vi "OP30A_Data.vi"() -> (0 "OP20_HOSE_TEST":T1)   [LabVIEW 2020]
panel:
  in  "[Constriction_Pr_Diff]":dbl
  in  "[Constriction_Act_Pr]":dbl
  in  "[Constriction_Diff_LL]":dbl
  in  "[Constriction_Diff_HL]":dbl
  in  "[Constriction_Result]":dbl
  in  "[Constriction_Test_Time]":dbl
  in  "[HP_STS]":dbl
  in  "[PRESSURE_FILL_ACT":dbl
  in  "[PRESSURE_DROP]":dbl
  in  "[PRESSURE_DROP_MAX]":dbl
  in  "[PRESSURE_FILL_LL]":dbl
  in  "[PRESSURE_FILL_HL]":dbl
  in  "[FILL_TIME]":dbl
  in  "[STAB_TIME]":dbl
  in  "[TEST_TIME]":dbl
  in  "[CT]":dbl
  out "error out":errorcluster
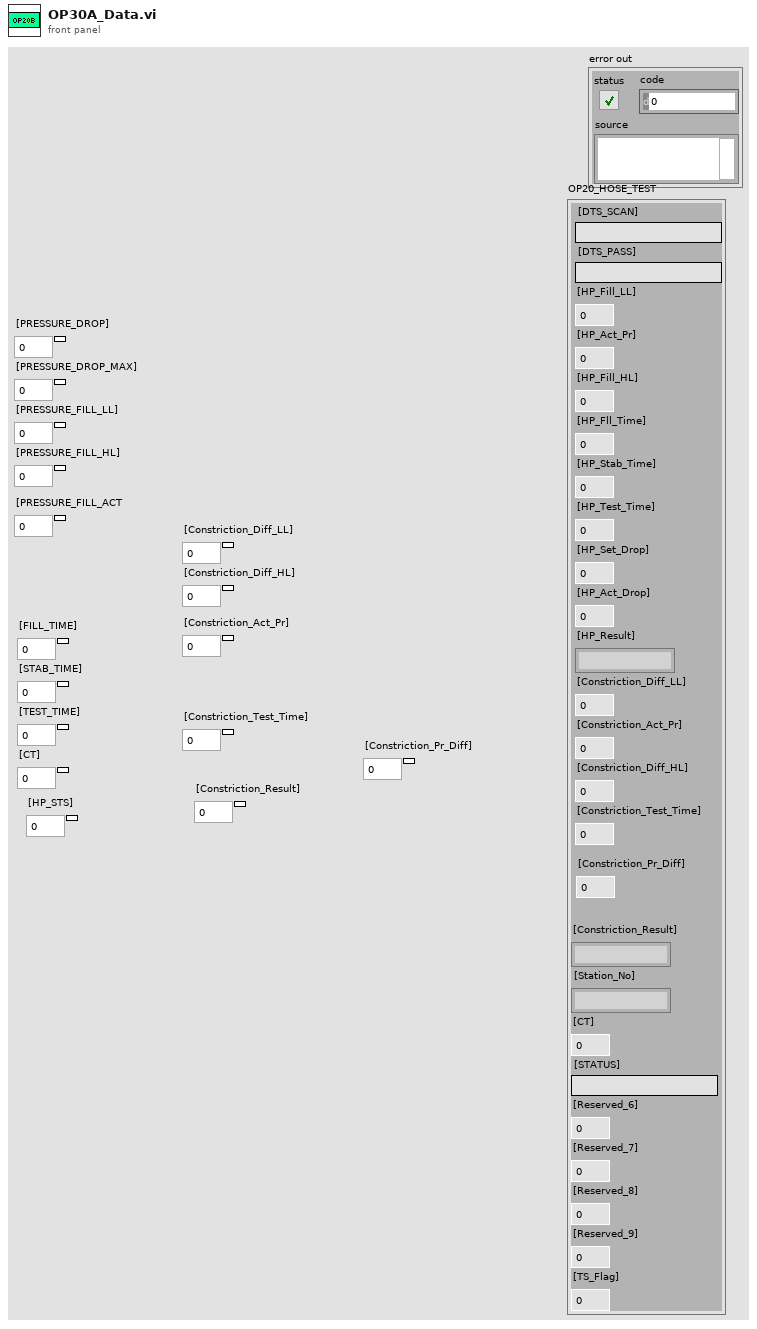
[diagram p1: front panel]
types:
  T1 = cluster{"[DTS_SCAN]":string, "[DTS_PASS]":string, "[HP_Fill_LL]":dbl, "[HP_Act_Pr]":dbl, "[HP_Fill_HL]":dbl, "[HP_Fll_Time]":dbl, "[HP_Stab_Time]":dbl, "[HP_Test_Time]":dbl, "[HP_Set_Drop]":dbl, "[HP_Act_Drop]":dbl, "[HP_Result]":string, "[Constriction_Diff_LL]":dbl, "[Constriction_Act_Pr]":dbl, "[Constriction_Diff_HL]":dbl, "[Constriction_Test_Time]":dbl, "[Constriction_Pr_Diff]":dbl, "[Constriction_Result]":string, "[Station_No]":string, "[CT]":dbl, "[STATUS]":string, "[Reserved_6]":dbl, "[Reserved_7]":dbl, "[Reserved_8]":dbl, "[Reserved_9]":dbl, "[TS_Flag]":dbl}
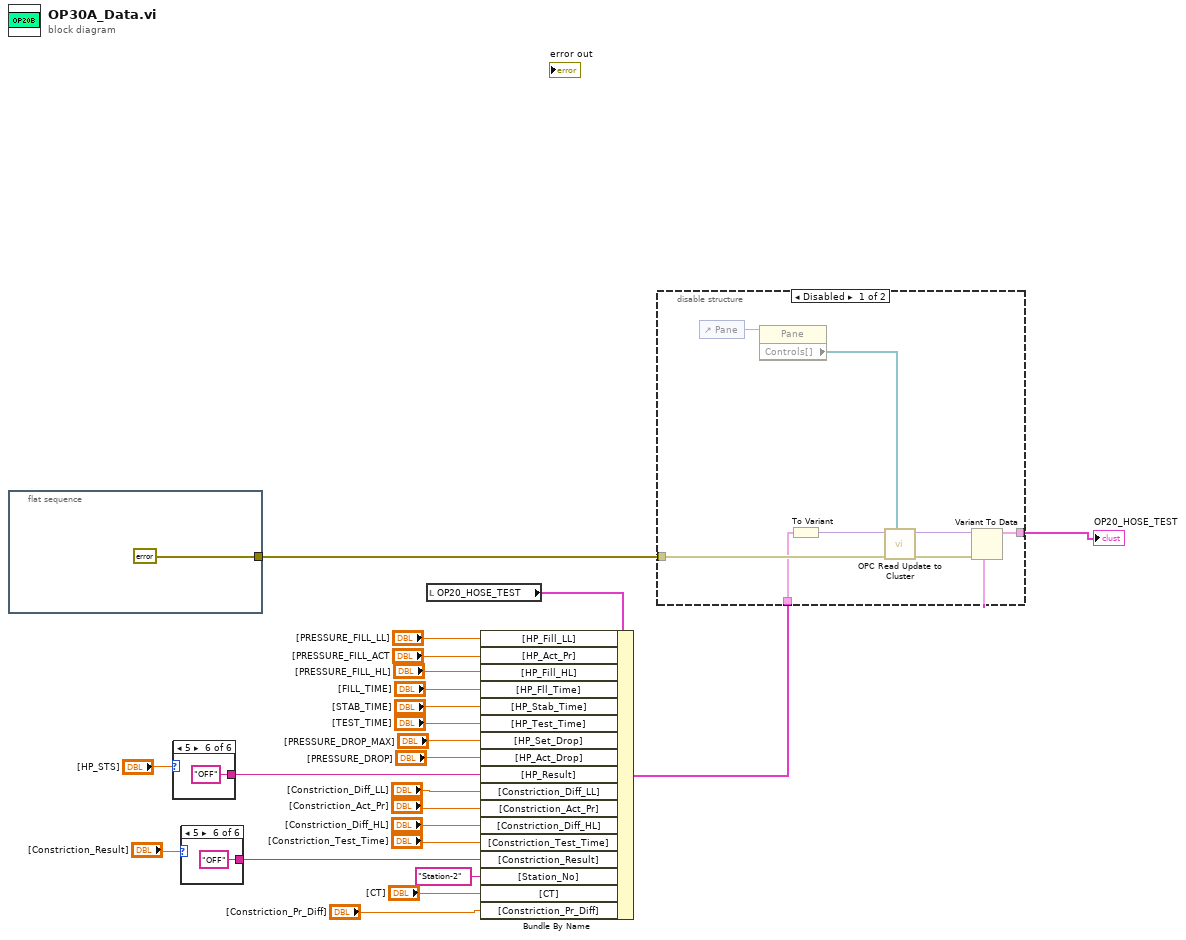
[diagram p0: block diagram]
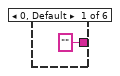
[diagram p2: hidden frame]
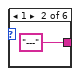
[diagram p3: hidden frame]
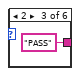
[diagram p4: hidden frame]
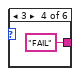
[diagram p5: hidden frame]
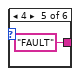
[diagram p6: hidden frame]
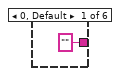
[diagram p7: hidden frame]
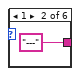
[diagram p8: hidden frame]
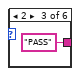
[diagram p9: hidden frame]
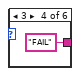
[diagram p10: hidden frame]
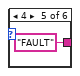
[diagram p11: hidden frame]
diagram:
  n1 = flat-sequence {
    tunnel: [errorcluster {"status"=FALSE, "code"=0, "source"=""} ("error in (no error)")] -> w23
    frame #0 {
    }
  }
  n2 = case shown="5" "[HP_STS]" {
    tunnel: ["" "---" "PASS" "FAIL" "FAULT" "OFF"] -> w11
    frame 0, Default {
    }
    frame 1 {
    }
    frame 2 {
    }
    frame 3 {
    }
    frame 4 {
    }
    frame 5 {
    }
  }
  n3 = case shown="5" "[Constriction_Result]" {
    tunnel: ["" "---" "PASS" "FAIL" "FAULT" "OFF"] -> w5
    frame 0, Default {
    }
    frame 1 {
    }
    frame 2 {
    }
    frame 3 {
    }
    frame 4 {
    }
    frame 5 {
    }
  }
  n4 = local read "OP20_HOSE_TEST"() -> (w22:T1)
  n5 = Bundle By Name(cluster=w22, "[HP_Fill_LL]"="[PRESSURE_FILL_LL]", "[HP_Act_Pr]"="[PRESSURE_FILL_ACT", "[HP_Fill_HL]"="[PRESSURE_FILL_HL]", "[HP_Fll_Time]"="[FILL_TIME]", "[HP_Stab_Time]"="[STAB_TIME]", "[HP_Test_Time]"="[TEST_TIME]", "[HP_Set_Drop]"="[PRESSURE_DROP_MAX]", "[HP_Act_Drop]"="[PRESSURE_DROP]", "[HP_Result]"=w11, "[Constriction_Diff_LL]"="[Constriction_Diff_LL]", "[Constriction_Act_Pr]"="[Constriction_Act_Pr]", "[Constriction_Diff_HL]"="[Constriction_Diff_HL]", "[Constriction_Test_Time]"="[Constriction_Test_Time]", "[Constriction_Result]"=w5, "[Station_No]"="Station-2", "[CT]"="[CT]", "[Constriction_Pr_Diff]"="[Constriction_Pr_Diff]") -> (w21:T1)
  n6 = disable-structure shown="Disabled" {
    disable-tunnel: w23 -> [w41 _]
    disable-tunnel: [w38 w45] -> w2
    disable-tunnel: w21 -> [w37 w45]
    frame Disabled {
      n7 = control-ref of="Pane"() -> (w40:refnum<vi>)
      n8 = property class="Pane"(reference=w40) -> ("Controls[]"=w39:refnum<vi>[])  [unwired: 1 in, 2 out]
      n9 = To Variant(anything=w37) -> (Variant=w42:variant)
      n10 = call "OPC Read Update to Cluster.vi"("Controls[]"=w39, "error in (no error)"=w41, "Variant in"=w42) -> ("error out"=w43:errorcluster, "Variant out"=w44:variant)  [unwired: 7 in]
      n11 = Variant To Data(error in=w43, type=w37, Variant=w44) -> (data=w38:T1)  [unwired: 1 out]
    }
    frame Enabled {
    }
  }
  "OP20_HOSE_TEST" <- w2
